vi "Digital Ouput Trigger.vi"(4 "MASTER in":T1 {"Image data"."Color Palette" items=["Grayscale U8", "False Color", "Overexposed"]; "Image data"."Exposure time [us]" format="%#_10g"; "Queue"."Initial time [s]" format="%_19f"; "Queue"."Raw data [V]\n(all samples)" format="%0.2f"; "Queue"."Timestamp [s]" format="%_19f"}) -> (1 "MASTER out":T1 {"Image data"."Color Palette" items=["Grayscale U8", "False Color", "Overexposed"]; "Image data"."Exposure time [us]" format="%#_10g"; "Queue"."Initial time [s]" format="%_19f"; "Queue"."Raw data [V]\n(all samples)" format="%0.2f"; "Queue"."Timestamp [s]" format="%_19f"}, 2 "Image count":dbl)   [LabVIEW 2020]
uses:
  MASTER.ctl
  Constants.ctl
  QBundle.ctl
  Queue.ctl
  Image data.ctl
  <vilib>/userdefined/High Color/IMAQdx.ctl
  <vilib>/vision/Image Controls.llb/IMAQ Image.ctl
  Image QBundle.ctl
  <vilib>/DAQmx/write.llb/DAQmx Write (Digital Bool 1Line 1Point).vi
  <vilib>/DAQmx/miscellaneous.llb/DAQmx Fill In Error Info.vi
panel:
  # "Description:\nWrites true, pause, false to digital output DAQmx task and increments image count when true."
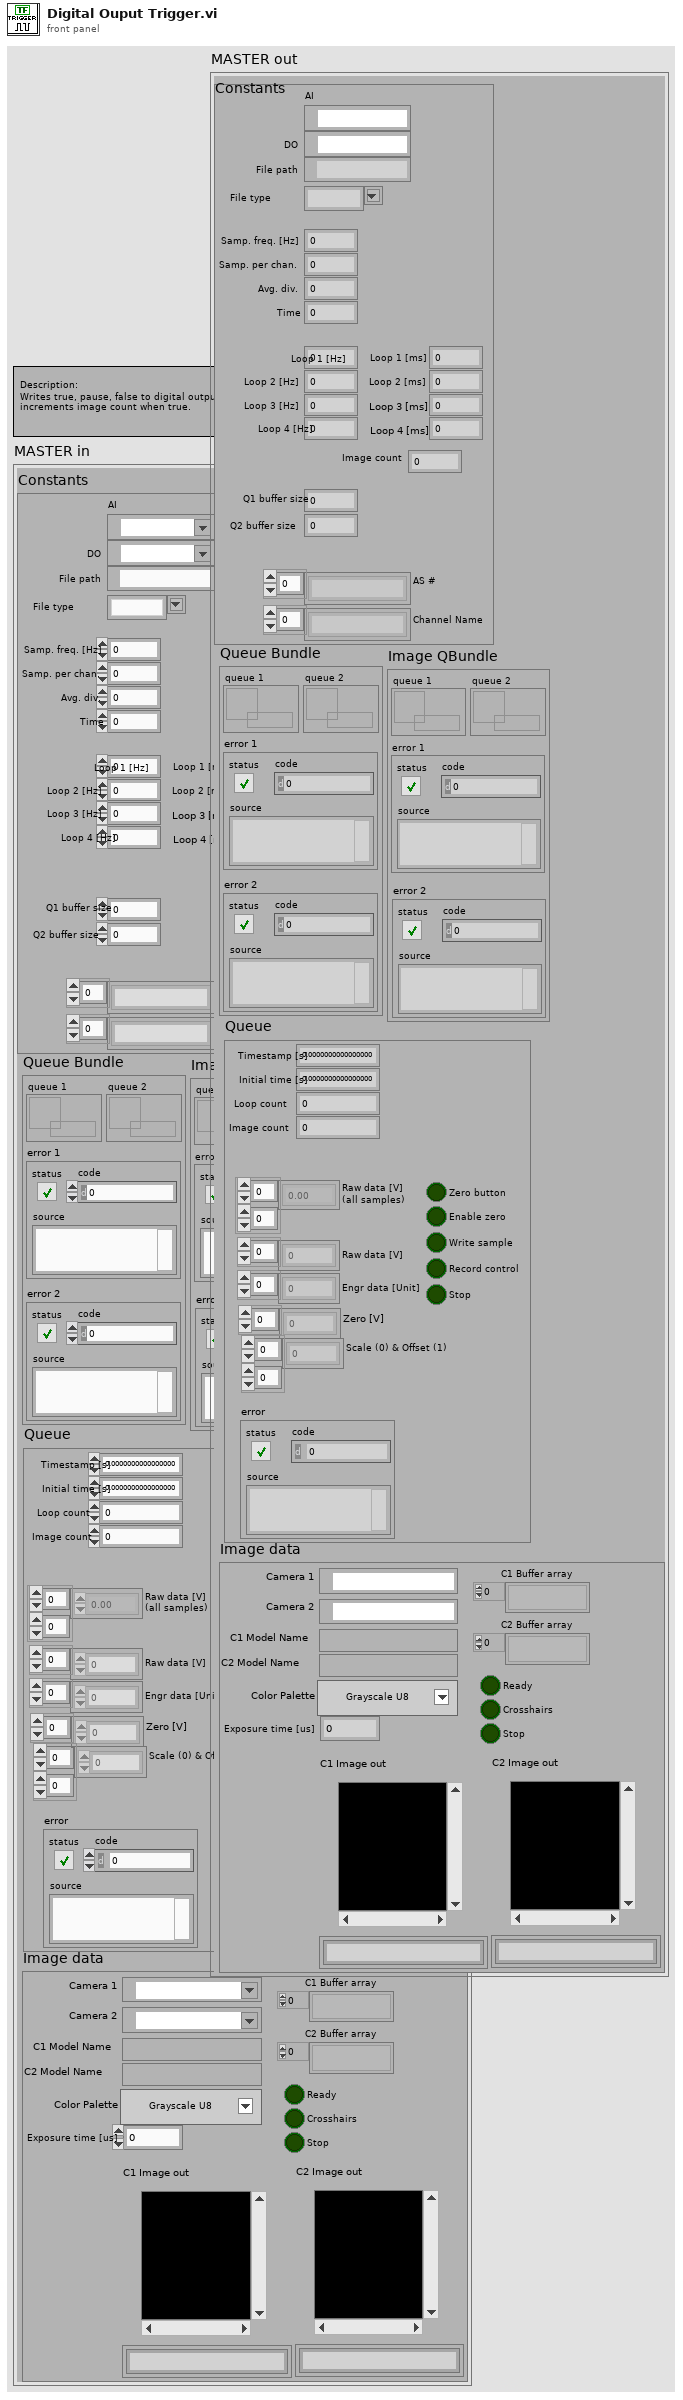
[diagram p1: front panel]
types:
  T1 = typedef "MASTER.ctl" = cluster{"Constants":T2, "Queue Bundle":T3, "Queue":T4, "Image data":T5, "Image QBundle ":T8}
  T2 = typedef "Constants.ctl" = cluster{"Time":u16, "Samp. freq. [Hz]":dbl, "Samp. per chan.":i32, "Avg. div.":i32, "File path":path, "AI":refnum<k21>, "Loop 1 [Hz]":dbl, "Loop 2 [Hz]":dbl, "Loop 3 [Hz]":dbl, "Loop 1 [ms]":dbl, "Loop 2 [ms]":dbl, "Loop 3 [ms]":dbl, "Q1 buffer size":i32, "Q2 buffer size":i32, "File type":string, "Loop 4 [Hz]":dbl, "Loop 4 [ms]":dbl, "Channel Name":string[], "AS #":string[], "DO":refnum<k21>}
  T3 = typedef "QBundle.ctl" = cluster{"queue 1":refnum<queue>, "error 1":errorcluster, "queue 2":refnum<queue>, "error 2":errorcluster}
  T4 = typedef "Queue.ctl" = cluster{"Enable zero":bool, "Engr data [Unit]":dbl[], "Zero button":bool, "Zero [V]":dbl[], "Timestamp [s]":dbl, "Write sample":bool, "Record control":bool, "Stop":bool, "error":errorcluster, "Raw data [V]\n(all samples)":dbl[][], "Raw data [V]":dbl[], "Loop count":i64, "Initial time [s]":dbl, "Scale (0) & Offset (1)":dbl[][], "Image count":dbl}
  T5 = typedef "Image data.ctl" = cluster{"Camera 1":T6, "Camera 2":T6, "C1 Image out ":T7, "C2 Image out":T7, "C1 Model Name":string, "C2 Model Name":string, "Exposure time [us]":dbl, "Color Palette":u16, "C1 Buffer array":T7[], "Ready":bool, "C2 Buffer array":T7[], "Crosshairs":bool, "Stop":bool}
  T6 = typedef "IMAQdx.ctl" = refnum<k21>
  T7 = typedef "IMAQ Image.ctl" = refnum<image>
  T8 = typedef "Image QBundle.ctl" = cluster{"queue 1":refnum<queue>, "error 1":errorcluster, "queue 2":refnum<queue>, "error 2":errorcluster}
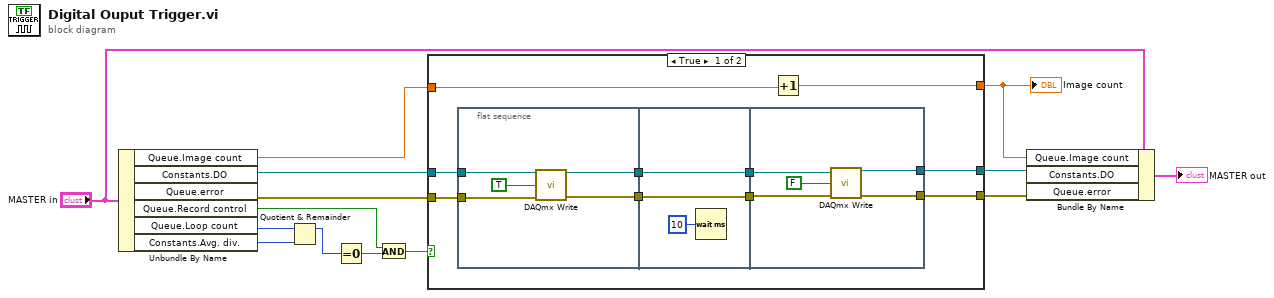
[diagram p0: block diagram]
diagram:
  n1 = Unbundle By Name("MASTER in") -> ("Queue.Image count"=w10:dbl, "Constants.DO"=w14:refnum<k21>, "Queue.error"=w13:errorcluster, "Queue.Record control"=w2:bool, "Queue.Loop count"=w5:i64, "Constants.Avg. div."=w4:i32)
  n2 = Quotient & Remainder(x=w5, y=w4) -> (x-y*floor(x/y)=w3:i64)  [unwired: 1 out]
  n3 = Equal To 0?(x=w3) -> (x = 0?=w1:bool)
  n4 = And(x=w2, y=w1) -> (x .and. y?=w6:bool)
  n5 = case shown="True" w6 {
    tunnel: w14 -> [w20 w40]
    tunnel: w13 -> [w19 w39]
    tunnel: [w18 w40] -> w12
    tunnel: [w17 w39] -> w7
    tunnel: w10 -> [w16 w38]
    tunnel: [w15 w38] -> w9
    frame True {
      n6 = flat-sequence {
        tunnel: [w29] -> w24
        tunnel: [w28] -> w23
        tunnel: w20 -> [w27]
        tunnel: w19 -> [w26]
        tunnel: w24 -> [w32]
        tunnel: w23 -> [w31]
        tunnel: [w32] -> w22
        tunnel: [w31] -> w21
        tunnel: w22 -> [w37]
        tunnel: w21 -> [w36]
        tunnel: [w35] -> w18
        tunnel: [w34] -> w17
        frame #0 {
          n7 = call-poly <vilib>:"DAQmx Write.vi"("task/channels in"=w27, "data"=TRUE, "error in"=w26) -> ("task out"=w29:refnum<k21>, "error out"=w28:errorcluster)  [unwired: 10 in, 1 out]
        }
        frame #1 {
          n8 = Wait (ms)(milliseconds to wait=u32 10) -> ()  [unwired: 1 out]
        }
        frame #2 {
          n9 = call-poly <vilib>:"DAQmx Write.vi"("task/channels in"=w37, "data"=FALSE, "error in"=w36) -> ("task out"=w35:refnum<k21>, "error out"=w34:errorcluster)  [unwired: 10 in, 1 out]
        }
      }
      n10 = Increment(x=w16) -> (x+1=w15:dbl)
    }
    frame False {
    }
  }
  "Image count" <- w9
  n11 = Bundle By Name(cluster="MASTER in", "Queue.Image count"=w9, "Constants.DO"=w12, "Queue.error"=w7) -> (→"MASTER out":T1)
